vi "Open from ProjFile.vi"(8 "error in (no error)":errorcluster, 10 "LV Project file path":path, 11 "LanguageData in":refnum<class "Project Data.lvclass">) -> (0 "error out":errorcluster, 3 "LanguageData out":refnum<class "Project Data.lvclass">)   [LabVIEW 2013, in "SET Project Data.lvlib" / "Project Data.lvclass"]
uses:
  Project Data.lvclass
  Project Data.lvclass/Project Data.ctl
  Resource Data Class/Resource Data.lvclass
  VI Class/VI Data.lvclass
  SET Project Data.lvlib
  Menu Class/Menu Data.lvclass
panel:
  # "Files must exist!"
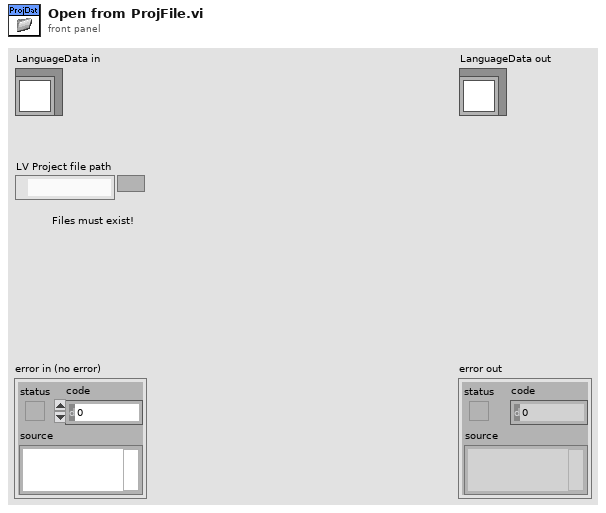
[diagram p1: front panel]
types:
  T1 = typedef "SET Project Data.lvlib/ProjFile_Resources Data.ctl" = cluster{"Languages []":T2[], "Resources []":T3[]}
  T2 = typedef "SET Project Data.lvlib/ProjFile_Language Entry.ctl" = cluster{"Tag":string, "Name":string, "Code Page":u16}
  T3 = typedef "SET Project Data.lvlib/ProjFile_Resource Entry.ctl" = cluster{"RID":string, "Tag":string, "Strings [] (UTF-16)":string[], "Shared?":bool}
  T4 = typedef "SET Project Data.lvlib/ProjFile_Project Data.ctl" = cluster{"Menu Data[]":T5[], "VI Data[]":T6[]}
  T5 = typedef "SET Project Data.lvlib/ProjFile_Menu Data.ctl" = cluster{"Menu Path":path, "Menu Items[]":cluster{"Tag":string, "RID":string}[]}
  T6 = typedef "SET Project Data.lvlib/ProjFile_VI Data.ctl" = cluster{"VI Path":path, "GObjects[]":T7[]}
  T7 = typedef "SET Project Data.lvlib/ProjFile_GObject Data.ctl" = cluster{"UID":i32, "Label":string, "ClassName":string, "Item List[]":cluster{"Item Name":string, "RID":string}[]}
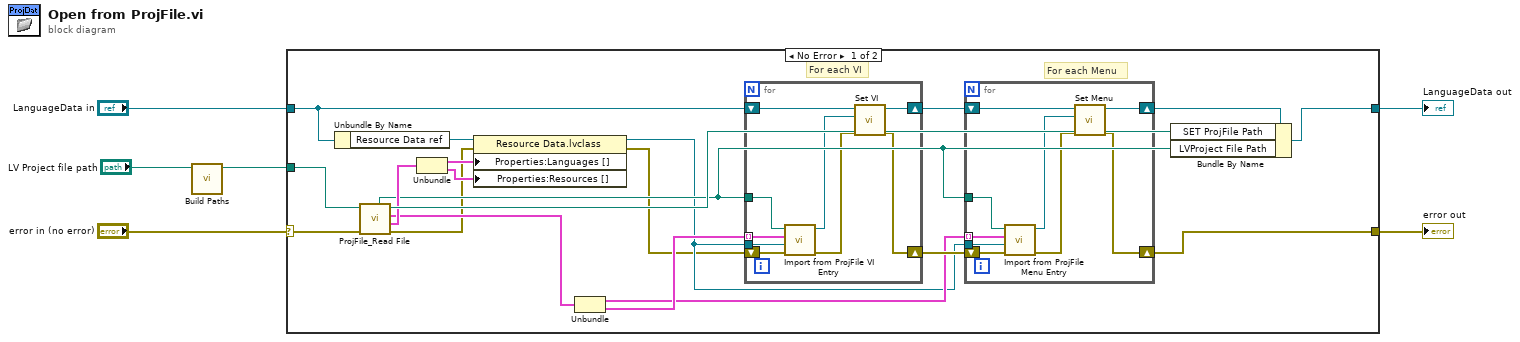
[diagram p0: block diagram]
diagram:
  n1 = call "Build Paths.vi"("lvproj Path"="LV Project file path") -> ("SET ProjFile Path"=w2:path)  [unwired: 10 in]
  n2 = case shown="No Error" "error in (no error)" {
    selector: "error in (no error)" -> [w26 w46]
    tunnel: [w18 w46] -> w5
    tunnel: [w15 w45] -> w4
    tunnel: "LanguageData in" -> [w23 w45]
    tunnel: w2 -> [w25 _]
    frame No Error {
      # "For each Menu"
      # "For each VI"
      n3 = Unbundle By Name(w23) -> ("Resource Data ref"=w12:refnum<data-value>)
      n4 = call "ProjFile_Read File.vi"("error in"=w26, "file (use dialog)"=w25) -> ("error out"=w8:errorcluster, "Resource Data"=w22:T1, "Project Data"=w21:T4, "LangData File Path"=w24:path, "Assumed Project Path"=w17:path)  [unwired: 5 in]
      n5 = Unbundle(w22) -> ("Languages []"=w10:T2[], "Resources []"=w9:T3[])
      n6 = property class="Resource Data.lvclass"(reference=w12, error in=w8, "Properties:Languages []"=w10, "Properties:Resources []"=w9) -> (reference out=w11:refnum<data-value>, error out=w7:errorcluster)
      n7 = Unbundle(w21) -> ("Menu Data[]"=w16:T5[], "VI Data[]"=w20:T6[])
      n8 = for {
        tunnel: w11 -> [w43]
        shift-right: [w38] -> w19
        shift-left: w7 -> [w44]
        shift-right: [w41] -> w14
        shift-left: w23 -> [w42]
        tunnel: w17 -> [w37]
        tunnel: w20 -> [w36] mode=indexing
        n9 = call "Import from ProjFile VI Entry.vi"("error in (no error)"=w44, "LangFile ref"=w43, "VI Data"=w36, "LVProject File Path (Absolute)"=w37) -> ("error out"=w39:errorcluster, "LanguageData out"=w40:refnum<class "VI Data.lvclass">)  [unwired: 6 in]
        n10 = call-dynamic "Set VI.vi"("error in (no error)"=w39, "VI Data in"=w40, "ProjectData in"=w42) -> ("error out"=w38:errorcluster, "ProjectData out"=w41:refnum<class "Project Data.lvclass">)  [unwired: 6 in, 1 out]
      }
      n11 = for {
        tunnel: w11 -> [w34]
        shift-right: [w29] -> w18
        shift-left: w19 -> [w35]
        shift-right: [w32] -> w13
        shift-left: w14 -> [w33]
        tunnel: w17 -> [w28]
        tunnel: w16 -> [w27] mode=indexing
        n12 = call "Import from ProjFile Menu Entry.vi"("error in (no error)"=w35, "LangFile ref"=w34, "Menu Data"=w27, "LVProject File Path"=w28) -> ("error out"=w30:errorcluster, "Menu Data out"=w31:refnum<class "Menu Data.lvclass">)  [unwired: 6 in]
        n13 = call-dynamic "Set Menu.vi"("error in (no error)"=w30, "RTM Data in"=w31, "ProjectData in"=w33) -> ("error out"=w29:errorcluster, "ProjectData out"=w32:refnum<class "Project Data.lvclass">)  [unwired: 6 in, 1 out]
      }
      n14 = Bundle By Name(cluster=w13, "SET ProjFile Path"=w24, "LVProject File Path"=w17) -> (w15:refnum<class "Project Data.lvclass">)
    }
    frame Error {
    }
  }
  "error out" <- w5
  "LanguageData out" <- w4
